vi "Store_Data.vi"(6 "Queues":T1, 8 "Status/Errors in":refnum<vi>, 10 "Write data parameters in":T2 caption="Data Storage" {"Data storage"."Detector number" format="%#.0f"}) -> ()   [LabVIEW 2013]
uses:
  Controls/Write_Data_Parameters.ctl
  Controls/Stop_Loop.ctl
  Controls/Data_Storage.ctl
  Controls/DB_Connection.ctl
  database/Connection.llb/Conn ObjectReference.ctl
  Controls/Data_Storage_Condition.ctl
  Controls/GPS_Timestamp.ctl
  Controls/Queues.ctl
  Controls/One_Second.ctl
  Controls/Get_Set_Statistics_Options2.ctl
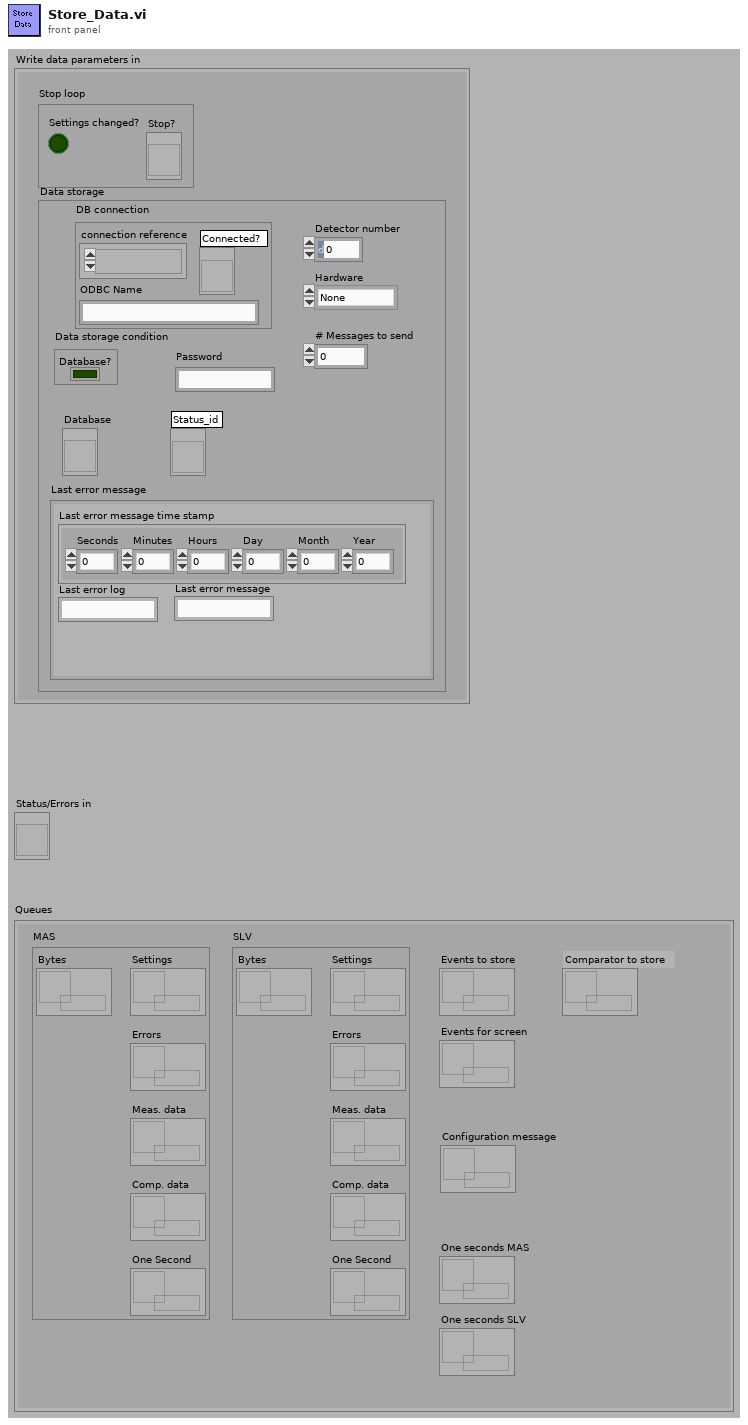
[diagram p1: front panel]
types:
  T1 = typedef "Queues.ctl" = cluster{"MAS":cluster{"Bytes":refnum<queue>, "Settings":refnum<queue>, "Errors":refnum<queue>, "Meas. data":refnum<queue>, "One Second":refnum<queue>, "Comp. data":refnum<queue>}, "SLV":cluster{"Bytes":refnum<queue>, "Settings":refnum<queue>, "Errors":refnum<queue>, "Meas. data":refnum<queue>, "One Second":refnum<queue>, "Comp. data":refnum<queue>}, "Events to store":refnum<queue>, "Events for screen":refnum<queue>, "One seconds MAS":refnum<queue>, "One seconds SLV":refnum<queue>, "Configuration message":refnum<queue>, "Comparator to store":refnum<queue>}
  T2 = typedef "Write_Data_Parameters.ctl" = cluster{"Stop loop":T3, "Data storage":T4}
  T3 = typedef "Stop_Loop.ctl" = cluster{"Settings changed?":bool, "Stop?":refnum<vi>}
  T4 = typedef "Data_Storage.ctl" = cluster{"DB connection":T5, "Data storage condition":T7, "Detector number":u16, "# Messages to send":i32, "Database":refnum<vi>, "Password":string, "Last error message":cluster{"Last error message time stamp":T8, "Last error log":string, "Last error message":string}, "Status_id":refnum<vi>, "Hardware":enum8{"None", "HiSPARC I", "HiSPARC II", "HiSPARC III", "Unknown"}}
  T5 = typedef "DB_Connection.ctl" = cluster{"connection reference":T6, "Connected?":refnum<vi>, "ODBC Name":string}
  T6 = typedef "Conn ObjectReference.ctl" = refnum<k1>
  T7 = typedef "Data_Storage_Condition.ctl" = cluster{"Database?":bool}
  T8 = typedef "GPS_Timestamp.ctl" = cluster{"Seconds":u8, "Minutes":u8, "Hours":u8, "Day":u8, "Month":u8, "Year":u16}
  T9 = typedef "Get_Set_Statistics_Options2.ctl" = enum16{"Get", "Set"}
  T10 = typedef "Rendezvous RefNum" = refnum<k1>
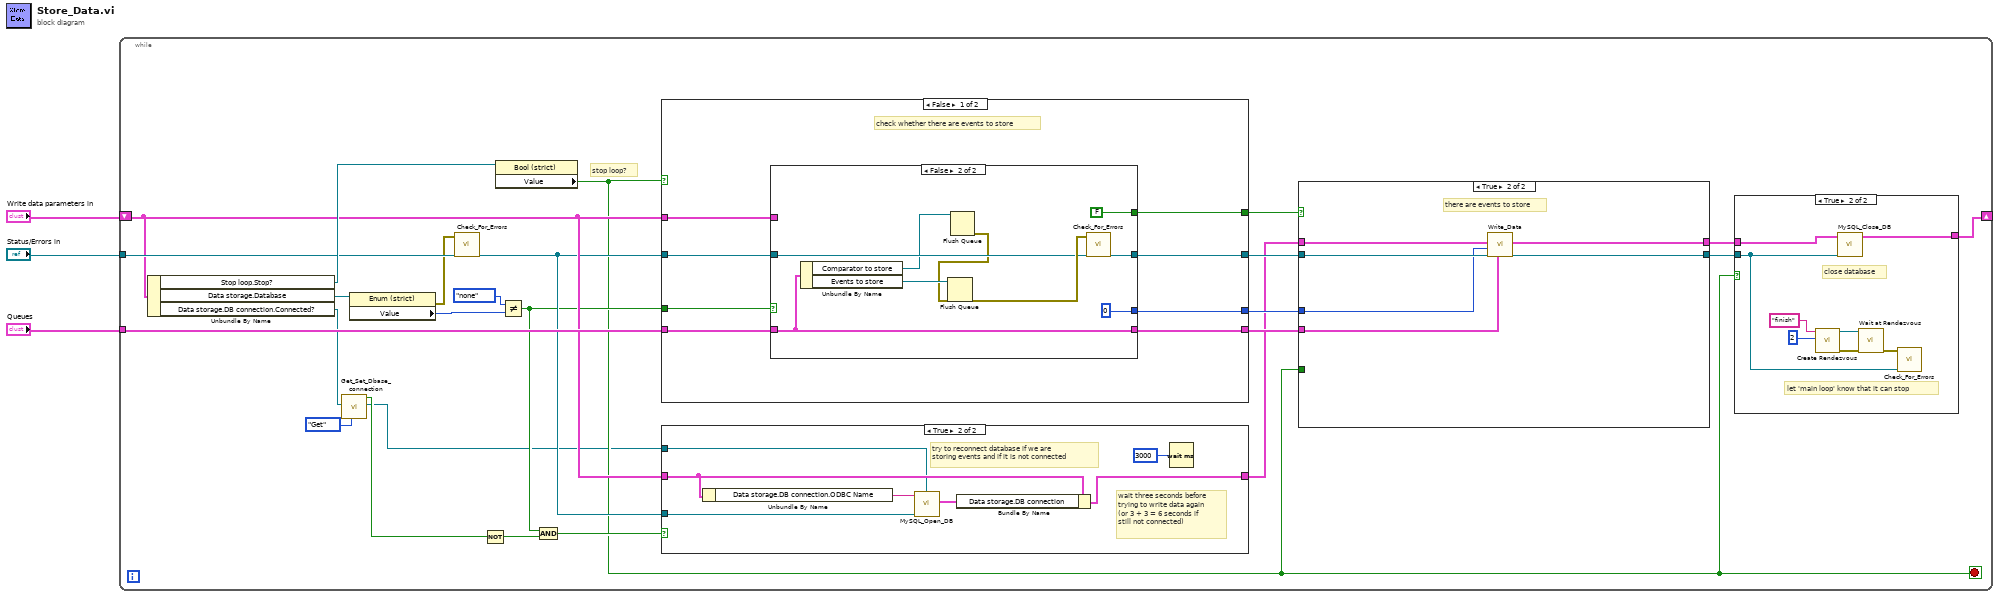
[diagram p0: block diagram]
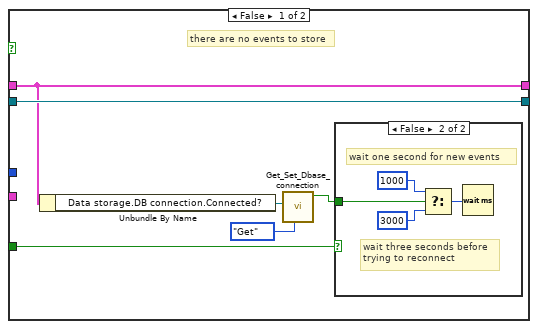
[diagram p3: hidden frame]
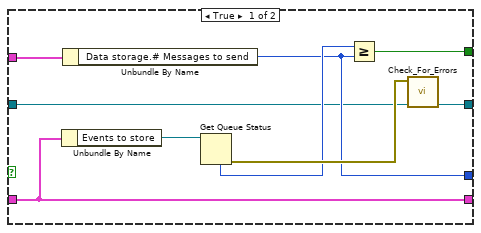
[diagram p6: hidden frame]
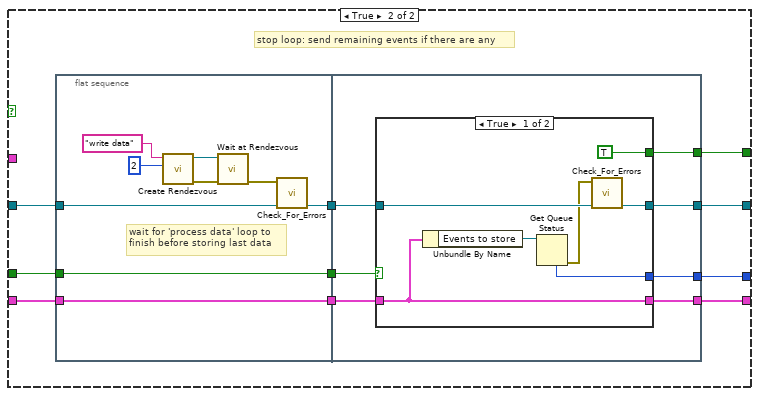
[diagram p7: hidden frame]
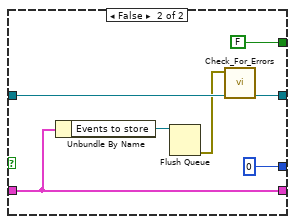
[diagram p8: hidden frame]
diagram:
  n1 = while {
    tunnel: "Status/Errors in" -> [w20]
    shift-right: [w27] -> _
    shift-left: "Write data parameters in" -> [w19]
    tunnel: "Queues" -> [w22]
    stop <- w8 stop-if-true
    # "stop loop?"
    n2 = Unbundle By Name(w19) -> ("Stop loop.Stop?"=w28:refnum<vi>, "Data storage.Database"=w14:refnum<vi>, "Data storage.DB connection.Connected?"=w7:refnum<vi>)
    n3 = call "Get_Set_Dbase_connection.vi"("Get/Set"=Get_Set_Statistics_Options2."Get", "Connected? in"=w7) -> ("Connected? out"=w4:refnum<vi>, "Value out"=w6:bool)  [unwired: 2 in, 6 out]
    n4 = property class="Enum (strict)"(reference=w14) -> (error out=w12:errorcluster, "Value"=w16:enum8{"none", "local", "central", "both"})  [unwired: 1 in, 1 out]
    n5 = call "Check_For_Errors.vi"("Status/Errors in"=w20, "error in"=w12) -> ("Status/Errors out"=w13:refnum<vi>)  [unwired: 9 out]
    n6 = Not(x=w6) -> (.not. x?=w9:bool)
    n7 = property class="Bool (strict)"(reference=w28) -> ("Value"=w8:bool)  [unwired: 1 in, 2 out]
    n8 = Not Equal?(x=enum8{"none", "local", "central", "both"}."none" ("Value"), y=w16) -> (x != y?=w10:bool)
    n9 = And(x=w10, y=w9) -> (x .and. y?=w11:bool)
    n10 = case shown="False" w8 {
      tunnel: w13 -> [w65 w94]
      tunnel: [w68 w95] -> w26
      tunnel: w19 -> [w67 _]
      tunnel: [w63 w88] -> w23
      tunnel: w22 -> [w69 w96]
      tunnel: [w64 w97] -> w17
      tunnel: [w66 w93] -> w21
      tunnel: w10 -> [w62 w90]
      frame False {
        # "check whether there are events to store"
        n11 = case shown="False" w62 {
          tunnel: w69 -> [w70 w83]
          tunnel: [w77 w86] -> w68
          tunnel: w67 -> [w75 _]
          tunnel: [w73 0 ("# Messages to send")] -> w66
          tunnel: w65 -> [w72 w84]
          tunnel: [w71 FALSE] -> w64
          tunnel: [w70 w83] -> w63
          frame True {
            n12 = Unbundle By Name(w70) -> ("Events to store"=w78:refnum<queue>)
            n13 = Unbundle By Name(w75) -> ("Data storage.# Messages to send"=w73:i32)
            n14 = Get Queue Status(queue=w78) -> (error out=w76:errorcluster, # elements in queue=w74:i32)  [unwired: 1 in, 7 out]
            n15 = Greater Or Equal?(x=w74, y=w73) -> (x >= y?=w71:bool)
            n16 = call "Check_For_Errors.vi"("Status/Errors in"=w72, "error in"=w76) -> ("Status/Errors out"=w77:refnum<vi>)  [unwired: 9 out]
          }
          frame False {
            n17 = Unbundle By Name(w83) -> ("Comparator to store"=w80:refnum<queue>, "Events to store"=w87:refnum<queue>)
            n18 = Flush Queue(queue=w80) -> (error out=w79:errorcluster)  [unwired: 1 in, 2 out]
            n19 = Flush Queue(queue=w87, error in (no error)=w79) -> (error out=w85:errorcluster)  [unwired: 2 out]
            n20 = call "Check_For_Errors.vi"("Status/Errors in"=w84, "error in"=w85) -> ("Status/Errors out"=w86:refnum<vi>)  [unwired: 9 out]
          }
        }
      }
      frame True {
        # "stop loop: send remaining events if there are any"
        n21 = flat-sequence {
          tunnel: w94 -> [w99]
          tunnel: w96 -> [w106]
          tunnel: [w106] -> w92
          tunnel: [w100] -> w91
          tunnel: w90 -> [w98]
          tunnel: [w98] -> w89
          tunnel: [w109] -> w97
          tunnel: [w112] -> w95
          tunnel: [w110] -> w93
          tunnel: w92 -> [w113]
          tunnel: w91 -> [w111]
          tunnel: w89 -> [w107]
          tunnel: [w108] -> w88
          frame #0 {
            # "wait for 'process data' loop to\nfinish before storing last data"
            n22 = call <vilib>:"Create Rendezvous.vi"("size (2)"=2, "name (unnamed)"="write data") -> ("error out"=w102:errorcluster, "rendezvous"=w101:T10)  [unwired: 1 in, 3 out]
            n23 = call <vilib>:"Wait at Rendezvous.vi"("error in (no error)"=w102, "rendezvous"=w101) -> ("error out"=w105:errorcluster)  [unwired: 1 in, 4 out]
            n24 = call "Check_For_Errors.vi"("Status/Errors in"=w99, "error in"=w105) -> ("Status/Errors out"=w100:refnum<vi>)  [unwired: 9 out]
          }
          frame #1 {
            n25 = case shown="True" w107 {
              tunnel: w113 -> [w114 w122]
              tunnel: [w119 w126] -> w112
              tunnel: w111 -> [w118 w125]
              tunnel: [w116 0 ("# elements in queue")] -> w110
              tunnel: [TRUE FALSE] -> w109
              tunnel: [w114 w122] -> w108
              frame True {
                n26 = Unbundle By Name(w114) -> ("Events to store"=w120:refnum<queue>)
                n27 = Get Queue Status(queue=w120) -> (error out=w117:errorcluster, # elements in queue=w116:i32)  [unwired: 1 in, 7 out]
                n28 = call "Check_For_Errors.vi"("Status/Errors in"=w118, "error in"=w117) -> ("Status/Errors out"=w119:refnum<vi>)  [unwired: 9 out]
              }
              frame False {
                n29 = Unbundle By Name(w122) -> ("Events to store"=w127:refnum<queue>)
                n30 = Flush Queue(queue=w127) -> (error out=w124:errorcluster)  [unwired: 1 in, 2 out]
                n31 = call "Check_For_Errors.vi"("Status/Errors in"=w125, "error in"=w124) -> ("Status/Errors out"=w126:refnum<vi>)  [unwired: 9 out]
              }
            }
          }
        }
      }
    }
    n32 = case shown="True" w11 {
      tunnel: w13 -> [_ w36]
      tunnel: w19 -> [w29 w32]
      tunnel: [w29 w34] -> w18
      tunnel: w4 -> [_ w30]
      frame False {
      }
      frame True {
        # "wait three seconds before\ntrying to write data again\n(or 3 + 3 = 6 seconds if\nstill not connected)"
        # "try to reconnect database if we are\nstoring events and if it is not connected"
        n33 = Unbundle By Name(w32) -> ("Data storage.DB connection.ODBC Name"=w31:string)
        n34 = call "MySQL_Open_DB.vi"("Connected? in"=w30, "Status/Errors in"=w36, "DB name"=w31) -> ("DB connection"=w35:T5)  [unwired: 2 in, 6 out]
        n35 = Bundle By Name(cluster=w32, "Data storage.DB connection"=w35) -> (w34:T2)
        n36 = Wait (ms)(milliseconds to wait=u32 3000 ("f")) -> ()  [unwired: 1 out]
      }
    }
    n37 = case shown="True" w17 {
      tunnel: w26 -> [w42 w51]
      tunnel: w18 -> [w41 w50]
      tunnel: [w41 w48] -> w24
      tunnel: [w42 w49] -> w25
      tunnel: w23 -> [_ w52]
      tunnel: w21 -> [_ w47]
      tunnel: w8 -> [w40 _]
      frame False {
        # "there are no events to store"
        n38 = Unbundle By Name(w41) -> ("Data storage.DB connection.Connected?"=w39:refnum<vi>)
        n39 = call "Get_Set_Dbase_connection.vi"("Get/Set"=Get_Set_Statistics_Options2."Get", "Connected? in"=w39) -> ("Value out"=w38:bool)  [unwired: 2 in, 7 out]
        n40 = case shown="False" w40 {
          tunnel: w38 -> [_ w44]
          frame True {
            # "don't wait and stop loop"
          }
          frame False {
            # "wait three seconds before\ntrying to reconnect"
            # "wait one second for new events"
            n41 = Select(t=u32 1000 ("milliseconds to wait"), s=w44, f=u32 3000) -> (s? t:f=w43:u32)
            n42 = Wait (ms)(milliseconds to wait=w43) -> ()  [unwired: 1 out]
          }
        }
      }
      frame True {
        # "there are events to store"
        n43 = call "Write_Data.vi"("Queues"=w52, "Status/Errors in"=w51, "# Events to store"=w47, "Write data parameters in"=w50) -> ("Status/Errors out"=w49:refnum<vi>, "Write data parameters out"=w48:T2)  [unwired: 6 out]
      }
    }
    n44 = case shown="True" w8 {
      tunnel: [w53 w54] -> w27
      tunnel: w24 -> [w53 w61]
      tunnel: w25 -> [_ w56]
      frame False {
      }
      frame True {
        # "let 'main loop' know that it can stop"
        # "close database"
        n45 = call <vilib>:"Create Rendezvous.vi"("size (2)"=2, "name (unnamed)"="finish") -> ("error out"=w59:errorcluster, "rendezvous"=w60:T10)  [unwired: 1 in, 3 out]
        n46 = call "MySQL_Close_DB.vi"("Status/Errors in"=w56, "Write Data Parameters in"=w61) -> ("Write Data Parameters out"=w54:T2)  [unwired: 1 in, 8 out]
        n47 = call <vilib>:"Wait at Rendezvous.vi"("error in (no error)"=w59, "rendezvous"=w60) -> ("error out"=w55:errorcluster)  [unwired: 1 in, 4 out]
        n48 = call "Check_For_Errors.vi"("Status/Errors in"=w56, "error in"=w55) -> ()  [unwired: 10 out]
      }
    }
  }
